vi "GEA2.vi"(0 "Connect Data":T2={"Com Port"=1, "Speed"=19200, "MyAddress"=128}, 2 "Function Call":T5(ring), 5 "Data_To_Send":T3={"pu8BufferToSend"=[128, 86], "u8TargetAddress"=96} {"u8TargetAddress" format="%.0x"}, 11 "error in (no error)":errorcluster) -> (4 "return type":i32, 6 "GetPendingMessage_Out":T4 {"pu8DataBufferToFill_Out" format="%.0x"}, 15 "error out":errorcluster)   [LabVIEW 2009]
uses:
  GEA2 Interface.dll
panel:
  out "pu8BufferToSend":u8[](array[numeric])
  out "pu8DataBufferToFillout":u8[](array[numeric])
  out "i32BufferSizeout":i32
  out "fMillisecondsout":dbl
  out "u32Secondsout":i32
  out "u32Minutesout":u32
  out "u32Hoursout":u32
  in  "DLL_IO_Parsed":T1(tab)
  out "u8Length":u8
  in  "u8Retries":u8=10
  in  "VISA resource name":refnum<visa-resource-name>
  in  "fMilliseconds":dbl
  in  "u32Seconds":i32
  in  "u32Minutes":u32
  in  "u32Hours":u32
  in  "pu8DataBufferToFill_In":u8[](array[numeric]) format="%.0x"
  # "Get Message Controls and Indicators"
  # "(Length is calculated from pu8Buffer to Send)"
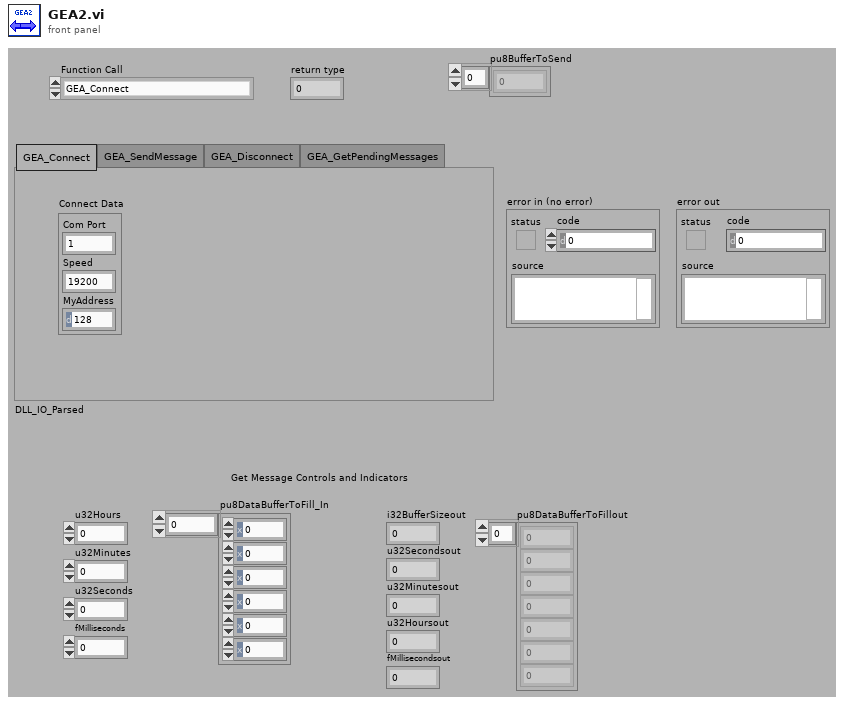
[diagram p1: front panel]
types:
  T1 = enum32{"GEA_Connect", "GEA_SendMessage", "GEA_Disconnect", "GEA_GetPendingMessages"}
  T2 = cluster{"Com Port":i32, "Speed":i32, "MyAddress":u8}
  T3 = cluster{"pu8BufferToSend":u8[], "u8TargetAddress":u8}
  T4 = cluster{"TimeStamp":string, "pu8DataBufferToFill_Out":u8[]}
  T5 = enum16{"GEA_Connect", "GEA_Disconnect", "GEA_GetPendingMessages", "GEA_SendMessage"}
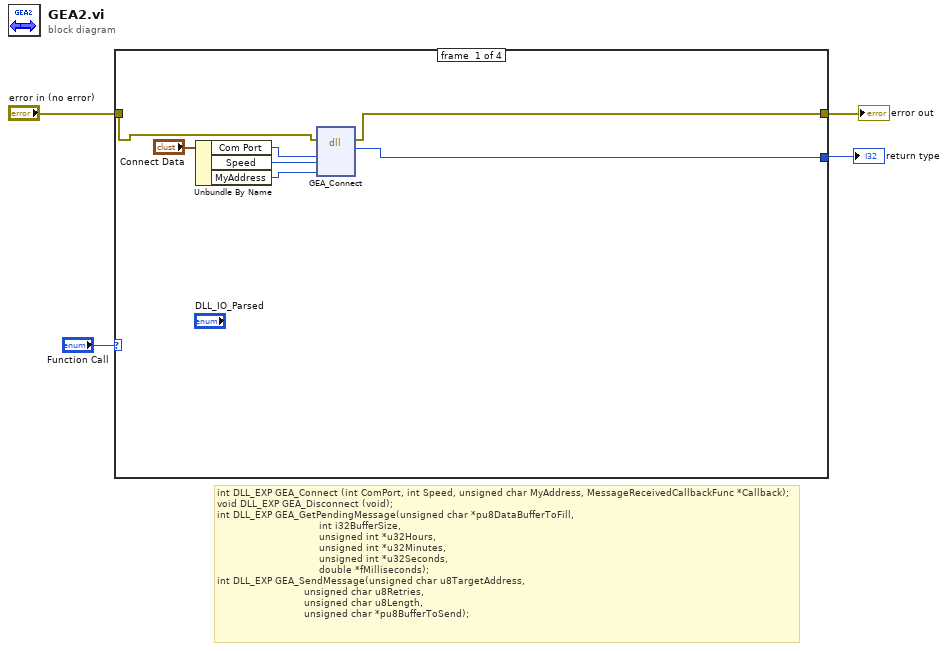
[diagram p0: block diagram]
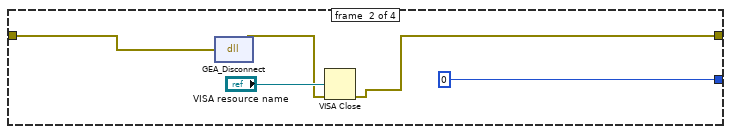
[diagram p2: hidden frame]
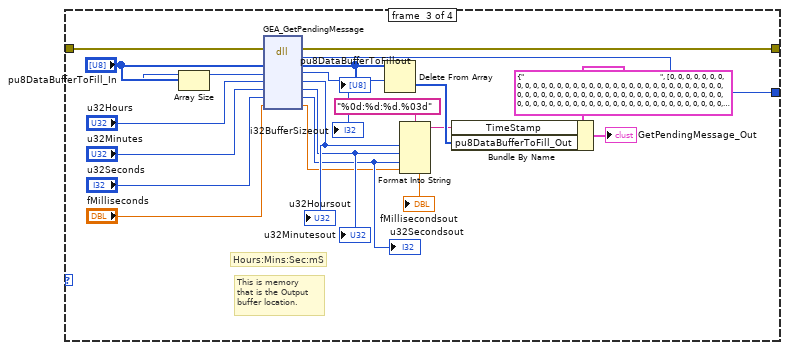
[diagram p3: hidden frame]
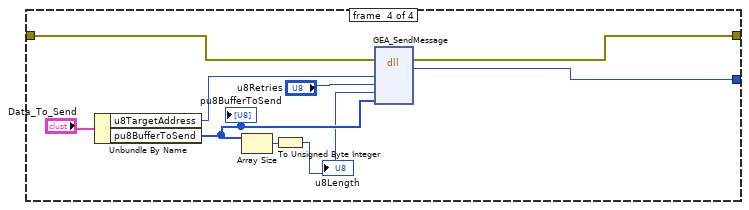
[diagram p4: hidden frame]
diagram:
  # "int DLL_EXP GEA_Connect (int ComPort, int Speed, unsigned char MyAddress, MessageReceivedCallbackFunc *Callback);\nvoid DLL_EXP GEA_Disconnect (void);\nint DLL_EXP GEA_GetPendingMessage(unsigned char *pu8DataBufferToFill, \n                                  int i32BufferSize, \n                                  unsigned int *u32Hours, \n                                  unsigned int *u32Minutes, \n                                  unsigned int *u32Seconds, \n                                  double *fMilliseconds);\nint DLL_EXP GEA_SendMessage(unsigned char u8TargetAddress, \n                             unsigned char u8Retries, \n                             unsigned char u8Length, \n                             unsigned char *pu8BufferToSend);"
  n1 = case shown="\"GEA_SendMessage\"" "Function Call" {
    tunnel: [w7 0 ("return type") w36 w44] -> w3
    tunnel: "error in (no error)" -> [w5 w15 w25 w39]
    tunnel: [w6 w12 w26 w38] -> w1
    frame #0 {
      n2 = Unbundle By Name("Connect Data") -> ("Com Port"=w10:i32, "Speed"=w9:i32, "MyAddress"=w8:u8)
      n3 = dll-call lib="C:/NI-2010/Trunk/Hybrid Water Heater/GEA2/GEA2 Interface.dll" fn="GEA_Connect"(error in=w5, "ComPort"=w10, "Speed"=w9, "MyAddress"=w8) -> (error out=w6:errorcluster, "return type"=w7:i32)  [unwired: 5 in, 1 out]
    }
    frame #1 {
      n4 = dll-call lib="C:/NI-2010/Trunk/Hybrid Water Heater/GEA2/GEA2 Interface.dll" fn="GEA_Disconnect"(error in=w15) -> (error out=w13:errorcluster)  [unwired: 3 in, 1 out]
      n5 = VISA Close(VISA resource name="VISA resource name", error in (no error)=w13) -> (error out=w12:errorcluster)
    }
    frame #2 {
      # "Hours:Mins:Sec:mS"
      # "This is memory\nthat is the Output\nbuffer location."
      n6 = Array Size(array="pu8DataBufferToFill_In") -> (size(s)=w17:i32)
      n7 = dll-call lib="C:/NI-2010/Trunk/Hybrid Water Heater/GEA2/GEA2 Interface.dll" fn="GEA_GetPendingMessage"(error in=w25, "pu8DataBufferToFill"="pu8DataBufferToFill_In", "i32BufferSize"=w17, "u32Hours"="u32Hours", "u32Minutes"="u32Minutes", "u32Seconds"="u32Seconds", "fMilliseconds"="fMilliseconds") -> (error out=w26:errorcluster, "return type"=w36:i32, "pu8DataBufferToFill"=w30:u8[], "i32BufferSize"=w29:i32, "u32Hours"=w34:u32, "u32Minutes"=w33:u32, "u32Seconds"=w32:i32, "fMilliseconds"=w31:dbl)  [unwired: 2 in, 1 out]
      "u32Hoursout" <- w34
      "u32Minutesout" <- w33
      "u32Secondsout" <- w32
      "fMillisecondsout" <- w31
      "i32BufferSizeout" <- w29
      "pu8DataBufferToFillout" <- w30
      n8 = Delete From Array(array=w30, length=w29) -> (deleted portion=w20:u8[])  [unwired: 1 in, 1 out]
      n9 = Format Into String(format string="%0d:%d:%d.%03d", w34, w33, w32, w31) -> (resulting string=w19:string)  [unwired: 2 in, 1 out]
      n10 = Bundle By Name(cluster=T4 {"TimeStamp"="                                                                    ", "pu8DataBufferToFill_Out"=[0, 0, 0, 0, 0, 0, 0, 0, 0, 0, 0, 0, 0, 0, 0, 0, 0, 0, 0, 0, 0, 0, 0, 0, 0, 0, 0, 0, 0, 0, 0, 0, 0, 0, 0, 0, 0, 0, 0, 0, 0, 0, 0, 0, 0, 0, 0, 0, 0, 0, 0, 0, 0, 0, 0, 0, 0, 0, 0, 0, 0, 0, 0, 0, 0, 0, 0, 0, 0, 0, 0, 0, 0, 0, 0, 0, 0, 0, 0, 0, 0, 0, 0, 0, 0, 0, 0, 0, 0, 0, 0, 0, 0, 0, 0, 0, 0, 0, 0, 0, 0, 0, 0, 0, 0, 0, 0, 0, 0, 0, 0, 0, 0, 0, 0, 0, 0, 0, 0, 0, 0, 0, 0, 0, 0, 0, 0, 0, 0, 0, 0, 0, 0, 0, 0, 0, 0, 0, 0, 0, 0, 0, 0, 0, 0, 0, 0, 0, 0, 0, 0, 0, 0, 0, 0, 0, 0, 0, 0, 0, 0, 0, 0, 0, 0, 0, 0, 0, 0, 0, 0, 0, 0, 0, 0, 0, 0, 0, 0, 0, 0, 0, 0, 0, 0, 0, 0, 0, 0, 0, 0, 0, 0, 0, 0, 0, 0, 0, 0, 0, 0, 0, 0, 0, 0, 0, 0, 0, 0, 0, 0, 0, 0, 0, 0, 0, 0, 0, 0, 0, 0, 0, 0, 0, 0, 0, 0, 0, 0, 0, 0, 0, 0, 0, 0, 0, 0, 0, 0, 0, 0, 0, 0, 0, 0, 0, 0, 0, 0, 0, 0, 0, 0, 0, 0, 0, 0, 0, 0, 0, 0, 0, 0, 0, 0, 0, 0, 0, 0, 0, 0, 0, 0, 0, 0, 0, 0, 0, 0, 0, 0, 0, 0, 0, 0, 0, 0, 0, 0, 0, 0, 0, 0, 0, 0, 0, 0, 0, 0, 0, 0, 0, 0, 0, 0, 0, 0, 0, 0, 0, 0, 0, 0, 0, 0, 0, 0, 0, 0, 0, 0, 0, 0, 0, 0, 0, 0, 0, 0, 0, 0, 0, 0, 0, 0, 0, 0, 0, 0, 0, 0, 0, 0, 0, 0, 0, 0, 0, 0, 0, 0, 0, 0, 0, 0, 0, 0, 0, 0, 0, 0, 0, 0, 0, 0, 0, 0, 0, 0, 0, 0, 0, 0, 0, 0, 0, 0, 0, 0, 0, 0, 0, 0, 0, 0, 0, 0, 0, 0, 0, 0, 0, 0, 0, 0, 0, 0, 0, 0, 0, 0, 0, 0, 0, 0, 0, 0, 0, 0, 0, 0, 0, 0, 0, 0, 0, 0, 0, 0, 0, 0, 0, 0, 0, 0, 0, 0, 0, 0, 0, 0, 0, 0, 0, 0, 0, 0, 0, 0, 0, 0, 0, 0, 0, 0, 0, 0, 0, 0, 0, 0, 0, 0, 0, 0, 0, 0, 0, 0, 0, 0, 0, 0, 0, 0, 0, 0, 0, 0, 0, 0, 0, 0, 0, 0, 0, 0, 0, 0, 0, 0, 0, 0, 0, 0, 0, 0, 0, 0, 0, 0, 0, 0, 0, 0, 0, 0, 0, 0, 0, 0, 0, 0, 0, 0, 0, 0, 0, 0, 0, 0, 0, 0]} ("GetPendingMessage_Out 3"), "TimeStamp"=w19, "pu8DataBufferToFill_Out"=w20) -> (→"GetPendingMessage_Out":T4)
    }
    frame #3 {
      n11 = Unbundle By Name("Data_To_Send") -> ("u8TargetAddress"=w41:u8, "pu8BufferToSend"=w40:u8[])
      "pu8BufferToSend" <- w40
      n12 = Array Size(array=w40) -> (size(s)=w43:i32)
      n13 = To Unsigned Byte Integer(number=w43) -> (unsigned 8bit integer=w37:u8)
      "u8Length" <- w37
      n14 = dll-call lib="C:/NI-2010/Trunk/Hybrid Water Heater/GEA2/GEA2 Interface.dll" fn="GEA_SendMessage"(error in=w39, "u8TargetAddress"=w41, "u8Retries"="u8Retries", "u8Length"=w37, "pu8BufferToSend"=w40) -> (error out=w38:errorcluster, "return type"=w44:i32)  [unwired: 6 in, 1 out]
    }
  }
  "return type" <- w3
  "error out" <- w1
